vi "GetServiceInfo.vi"(8 "error in (no error)":errorcluster, 11 "GRPCService in":refnum<class "GRPCService.lvclass">) -> (0 "error out":errorcluster, 2 "Service":T1, 3 "GRPCService out":refnum<class "GRPCService.lvclass">)   [LabVIEW 2019, in "MicronGRPCServer.lvlib" / "GRPCService.lvclass"]
uses:
  GRPCService.lvclass
  Base/Server/Service/Typedefs/MicronArgs.ctl
  GRPCService.lvclass/GRPCService.ctl
  Base/Server/Service/ServiceBase.lvclass
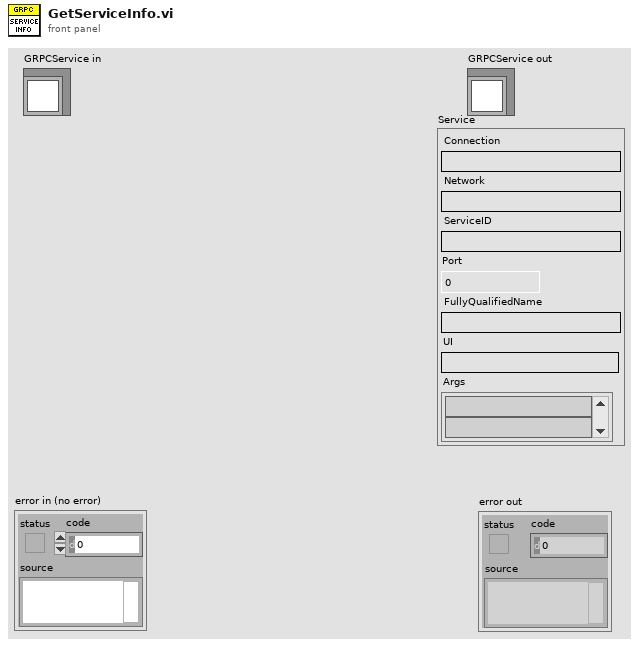
[diagram p1: front panel]
types:
  T1 = typedef "MicronServer.lvlib/ServiceBase.lvclass/MicronArgs.ctl" = cluster{"Connection":string, "Network":string, "ServiceID":string, "Port":i32, "FullyQualifiedName":string, "UI":string, "Args":string[]}
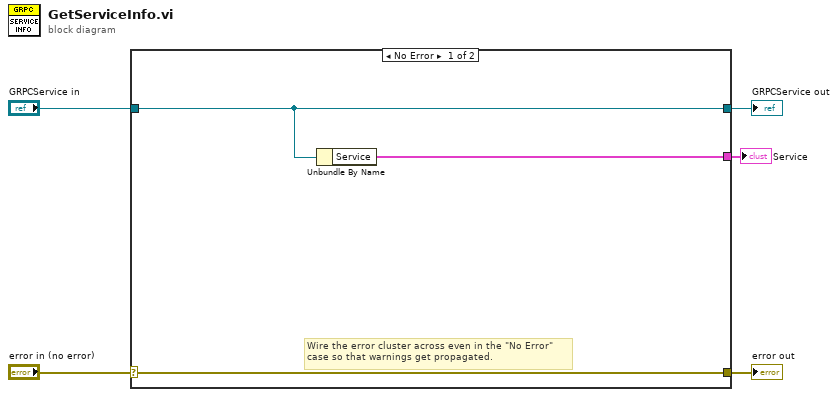
[diagram p0: block diagram]
diagram:
  n1 = case shown="No Error" "error in (no error)" {
    selector: "error in (no error)" -> [w8 w10]
    tunnel: [w8 w10] -> w4
    tunnel: [w7 w9] -> w2
    tunnel: "GRPCService in" -> [w7 w9]
    tunnel: [w6 _] -> w1
    frame No Error {
      # "Wire the error cluster across even in the \"No Error\"\ncase so that warnings get propagated."
      n2 = Unbundle By Name(w7) -> ("Service"=w6:T1)
    }
    frame Error {
    }
  }
  "error out" <- w4
  "GRPCService out" <- w2
  "Service" <- w1
